vi "sub_agv_main.vi"(8 "error in":errorcluster) -> (0 "error out":errorcluster)   [LabVIEW 2019]
panel:
  out "loop":i32
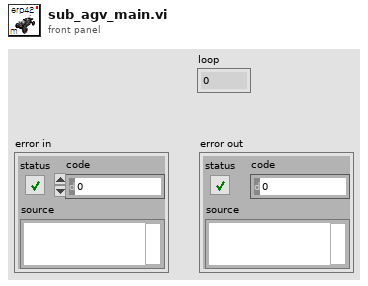
[diagram p1: front panel]
types:
  T1 = typedef "status.ctl" = u16
  T2 = cluster{"AGV":T1, "AGV Estop":T1, "Obstacle":T1, "Heading":T1, "Waypt":T1, "GNSS":T1, "VLP16":T1, "Cam":T1, "RPLidar":T1, "Joystick":T1}
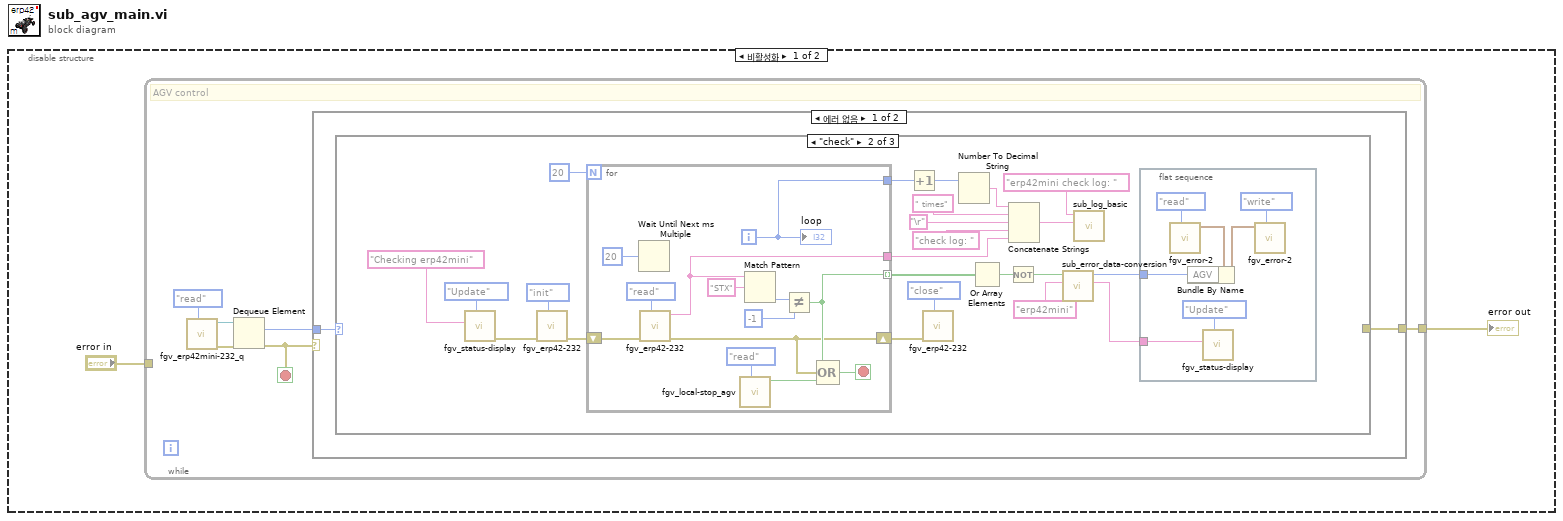
[diagram p0: block diagram]
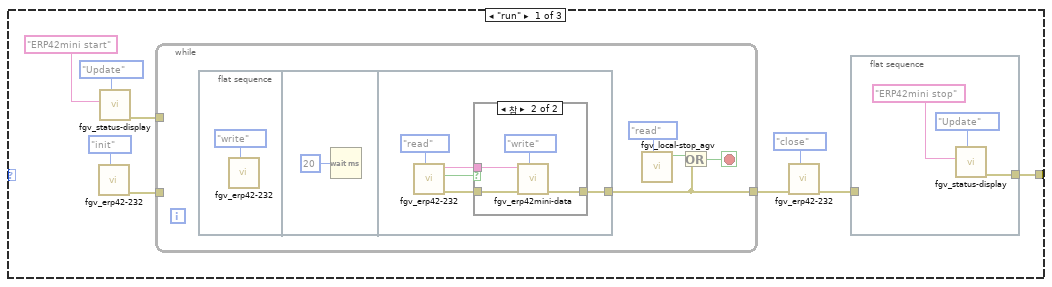
[diagram p2: hidden frame]
diagram:
  n1 = disable-structure shown="비활성화" {
    frame Disabled {
      n2 = while {
        tunnel: "error in" -> [_]
        tunnel: [w3] -> w1
        stop <- w4 stop-if-true
        # "AGV control"
        n3 = call "fgv_erp42mini-232_q.vi"("cmd"=enum16{"create", "write", "read", "close"}."read") -> ("error out"=w7:errorcluster, "queue out"=w6:refnum<queue>)  [unwired: 9 in]
        n4 = Dequeue Element(queue=w6, error in (no error)=w7) -> (element=w5:enum16{"run", "check", "stop"}, error out=w4:errorcluster)  [unwired: 1 in, 2 out]
        n5 = case shown="에러 없음" w4 {
          tunnel: w5 -> [w10 _]
          tunnel: [w9 _] -> w3
          frame No Error {
            n6 = case shown="\"check\"" w10 {
              tunnel: [w11 _ _] -> w9
              frame "run" {
                n7 = call "fgv_erp42-232.vi"("cmd"=enum16{"init", "read", "write", "close"}."init") -> ("error out"=w18:errorcluster)  [unwired: 8 in, 2 out]
                n8 = call "fgv_status-display.vi"("Mode"=enum16{"Initial", "Update", "Clear"}."Update", "title"="ERP42mini start" ("String in")) -> ("error out"=w12:errorcluster)  [unwired: 9 in]
                n9 = while {
                  tunnel: w18 -> [_]
                  tunnel: [w23] -> w15
                  tunnel: w12 -> [_]
                  stop <- w21 stop-if-true
                  n10 = flat-sequence {
                    tunnel: [w26] -> w23
                    frame #0 {
                      n11 = call "fgv_erp42-232.vi"("cmd"=enum16{"init", "read", "write", "close"}."write") -> ()  [unwired: 8 in, 3 out]
                    }
                    frame #1 {
                      n12 = Wait (ms)(milliseconds to wait=u32 20 ("ms 배수")) -> ()  [unwired: 1 out]
                    }
                    frame #2 {
                      n13 = call "fgv_erp42-232.vi"("cmd"=enum16{"init", "read", "write", "close"}."read") -> ("error out"=w27:errorcluster, "valid"=w29:bool, "read_buffer"=w28:string)  [unwired: 8 in]
                      n14 = case shown="참" w29 {
                        tunnel: w28 -> [_ w34]
                        tunnel: w27 -> [w31 w33]
                        tunnel: [w31 w32] -> w26
                        frame False {
                        }
                        frame True {
                          n15 = call "fgv_erp42mini-data.vi"("cmd"=enum16{"ini", "write", "read"}."write", "error in"=w33, "erp_read-data"=w34) -> ("error out"=w32:errorcluster)  [unwired: 7 in, 1 out]
                        }
                      }
                    }
                  }
                  n16 = call "fgv_local-stop_agv.vi"("cmd"=enum16{"ini", "read", "stop"}."read") -> ("stop status"=w22:bool)  [unwired: 10 in]
                  n17 = Or(x=w22, y=w23) -> (x .or. y?=w21:bool)
                }
                n18 = call "fgv_erp42-232.vi"("cmd"=enum16{"init", "read", "write", "close"}."close", "error in"=w15) -> ("error out"=w16:errorcluster)  [unwired: 7 in, 2 out]
                n19 = flat-sequence {
                  tunnel: w16 -> [_]
                  tunnel: [w36] -> w11
                  frame #0 {
                    n20 = call "fgv_status-display.vi"("Mode"=enum16{"Initial", "Update", "Clear"}."Update", "title"="ERP42mini stop" ("String in")) -> ("error out"=w36:errorcluster)  [unwired: 9 in]
                  }
                }
              }
              frame "check" {
                n21 = call "fgv_status-display.vi"("Mode"=enum16{"Initial", "Update", "Clear"}."Update", "title"="Checking erp42mini" ("String in")) -> ("error out"=w53:errorcluster)  [unwired: 9 in]
                n22 = call "fgv_erp42-232.vi"("cmd"=enum16{"init", "read", "write", "close"}."init", "error in"=w53) -> ("error out"=w59:errorcluster)  [unwired: 7 in, 2 out]
                n23 = for {
                  N: 20 -> [_]
                  tunnel: [w73] -> w56 mode=indexing
                  shift-right: [w70] -> w57
                  shift-left: w59 -> [w81]
                  tunnel: [w74] -> w41
                  tunnel: [w69] -> w44
                  i -> [w69]
                  stop <- w71 stop-if-true
                  n24 = Wait Until Next ms Multiple(millisecond multiple=u32 20 ("milliseconds to wait")) -> ()  [unwired: 1 out]
                  n25 = call "fgv_erp42-232.vi"("cmd"=enum16{"init", "read", "write", "close"}."read", "error in"=w81) -> ("error out"=w70:errorcluster, "read_buffer"=w74:string)  [unwired: 7 in, 1 out]
                  n26 = call "fgv_local-stop_agv.vi"("cmd"=enum16{"ini", "read", "stop"}."read") -> ("stop status"=w72:bool)  [unwired: 10 in]
                  n27 = Match Pattern(string=w74, regular expression="STX") -> (offset past match=w77:i32)  [unwired: 1 in, 3 out]
                  n28 = Not Equal?(x=w77, y=-1) -> (x != y?=w73:bool)
                  n29 = Compound Arithmetic op=OR ("복합 연산")(w73, w70, w72) -> (w71:bool)
                  "loop" <- w69
                }
                n30 = Increment(x=w44) -> (x+1=w47:i32)
                n31 = call "fgv_erp42-232.vi"("cmd"=enum16{"init", "read", "write", "close"}."close", "error in"=w57) -> ()  [unwired: 7 in, 3 out]
                n32 = Number To Decimal String(number=w47) -> (decimal integer string=w46:string)  [unwired: 1 in]
                n33 = Or Array Elements(Boolean array=w56) -> (logical OR=w49:bool)
                n34 = Not(x=w49) -> (.not. x?=w48:bool)
                n35 = Concatenate Strings(w46, " times" ("문자열"), "\r", "check log: " ("문자열"), w41) -> (w40:string)
                n36 = call "sub_error_data-conversion.vi"("name"="erp42mini", "error status"=w48) -> ("check result string"=w51:string, "error conversion out"=w52:T1)  [unwired: 8 in]
                n37 = call "sub_log_basic.vi"("desc"=w40, "Title"="erp42mini check log: ") -> ()  [unwired: 9 in, 1 out]
                n38 = flat-sequence {
                  tunnel: w52 -> [w68]
                  tunnel: w51 -> [w62]
                  frame #0 {
                    n39 = call "fgv_error-2.vi"("cmd"=enum16{"init", "read", "write"}."read") -> ("Error cluster out"=w67:T2)  [unwired: 9 in, 1 out]
                    n40 = Bundle By Name(cluster=w67, "AGV"=w68) -> (w66:T2)
                    n41 = call "fgv_status-display.vi"("Mode"=enum16{"Initial", "Update", "Clear"}."Update", "title"=w62) -> ()  [unwired: 9 in, 1 out]
                    n42 = call "fgv_error-2.vi"("cmd"=enum16{"init", "read", "write"}."write", "Error cluster"=w66) -> ()  [unwired: 8 in, 2 out]
                  }
                }
              }
              frame "stop", Default {
              }
            }
          }
          frame Error {
          }
        }
      }
      "error out" <- w1
    }
    frame Enabled {
    }
  }
